vi "Get Cell.vi"(8 "error in (no error)":errorcluster, 11 "Cell Context in":refnum<class "Cell Context.lvclass">) -> (0 "error out":errorcluster, 2 "Cell":refnum<class "Cell.lvclass">, 3 "Cell Context out":refnum<class "Cell Context.lvclass">)   [LabVIEW 2024, in "SourceGrid.lvlib" / "Cell Context.lvclass"]
uses:
  Cell Context.lvclass
  Cell Context.lvclass/Cell Context.ctl
  D:/git/Sourcegrid-LabVIEW/dll/SourceGrid.dll
  dll/SourceGrid.dll
  Cell/Cell.lvclass
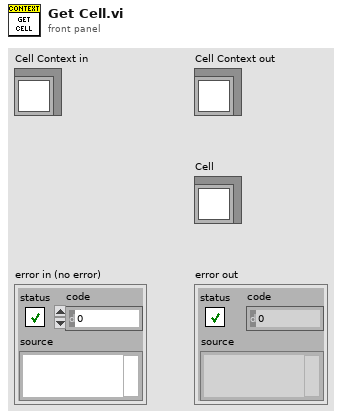
[diagram p1: front panel]
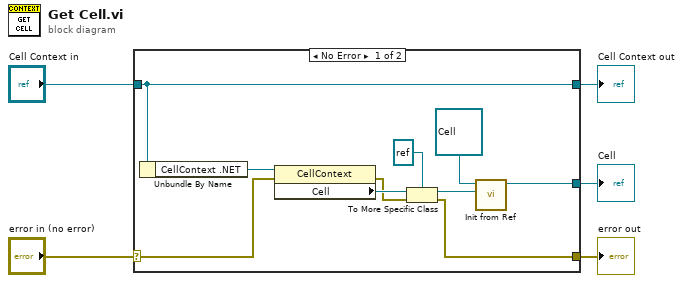
[diagram p0: block diagram]
diagram:
  n1 = case shown="No Error" "error in (no error)" {
    selector: "error in (no error)" -> [w13 w16]
    tunnel: [w7 w16] -> w4
    tunnel: [w15 w17] -> w2
    tunnel: "Cell Context in" -> [w15 w17]
    tunnel: [w6 _] -> w1
    frame No Error {
      n2 = Unbundle By Name(w15) -> ("CellContext .NET"=w14:refnum<k24>)
      n3 = property class="CellContext"(reference=w14, error in=w13) -> (error out=w8:errorcluster, "Cell"=w12:refnum<k24>)  [unwired: 1 out]
      n4 = To More Specific Class(target class=refnum<k24> refnum ("Cell Ref"), reference=w12, error in=w8) -> (specific class reference=w10:refnum<k24>, error out=w7:errorcluster)
      n5 = call-dynamic "Init from Ref.vi"("Cell Ref"=w10, "Cell in"=refnum<class "Cell.lvclass"> refnum) -> ("Cell out"=w6:refnum<class "Cell.lvclass">)  [unwired: 9 in]
    }
    frame Error {
    }
  }
  "error out" <- w4
  "Cell Context out" <- w2
  "Cell" <- w1
